vi "Client_Init.vi"(0 "object in":refnum<class "Client.lvclass">, 2 "File Type":T2, 3 "File Method":T1, 5 "Error In":errorcluster) -> (14 "object out":refnum<class "Client.lvclass">, 19 "Error Out":errorcluster)   [LabVIEW 2024, in "Client.lvclass"]
uses:
  Client.lvclass
  Support/Type Def/File Type.ctl
  Support/Type Def/File Method.ctl
  Implementations/Logger/Logger.lvclass
  Implementations/Viewer/Viewer.lvclass
  Abstractions/Excel/Excel.lvclass
  Abstractions/TDMS/TDMS.lvclass
  Client.lvclass/Client.ctl
  <vilib>/Utility/file.llb/Write Delimited Spreadsheet (string).vi
  IDataMethod_interface/IDataMethod.lvclass
  Abstractions/DataType/DataType.lvclass
panel:
  # "Connector Pane"
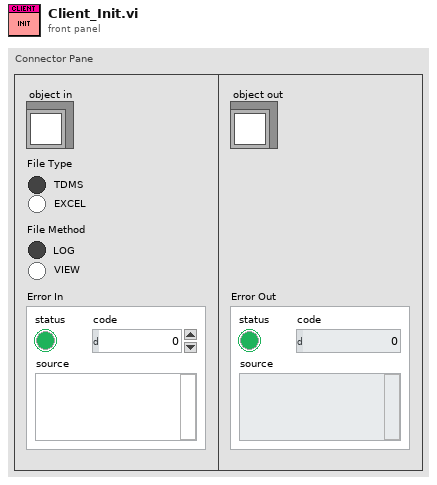
[diagram p1: front panel]
types:
  T1 = typedef "File Method.ctl" = enum32{"Log", "View"}
  T2 = typedef "File Type.ctl" = enum32{"TDMS", "EXCEL"}
  T3 = enum16{"open", "open or create", "create or replace", "create", "open (read-only)"}
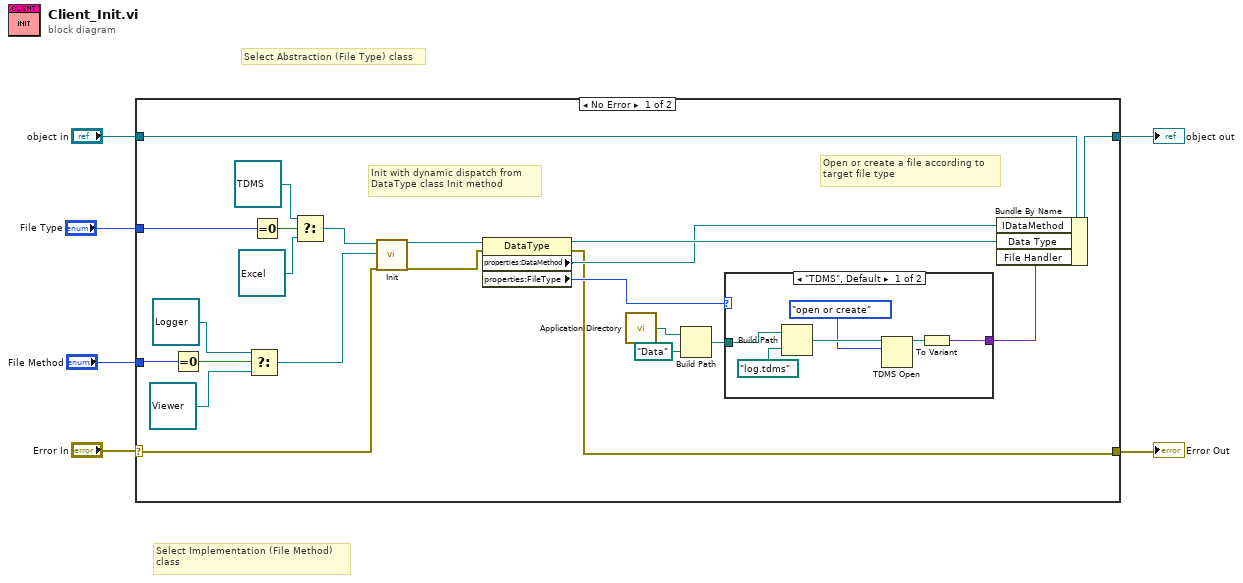
[diagram p0: block diagram]
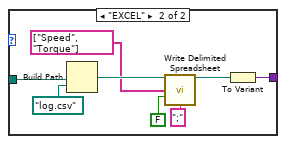
[diagram p2: hidden frame]
diagram:
  # "Select Abstraction (File Type) class"
  # "Select Implementation (File Method)\nclass"
  n1 = case shown="No Error" "Error In" {
    selector: "Error In" -> [w10 w44]
    tunnel: "object in" -> [w29 w45]
    tunnel: [w28 w45] -> w5
    tunnel: [w20 w44] -> w3
    tunnel: "File Method" -> [w19 _]
    tunnel: "File Type" -> [w16 _]
    frame No Error {
      # "Open or create a file according to\ntarget file type"
      # "Init with dynamic dispatch from\nDataType class Init method"
      n2 = Equal To 0?(x=w19) -> (x = 0?=w18:bool)
      n3 = Select(t=refnum<class "Logger.lvclass"> refnum ("Logger"), s=w18, f=refnum<class "Viewer.lvclass"> refnum ("Viewer")) -> (s? t:f=w11:refnum<class "IDataMethod.lvclass">)
      n4 = Equal To 0?(x=w16) -> (x = 0?=w17:bool)
      n5 = Select(t=refnum<class "TDMS.lvclass"> refnum ("TDMS"), s=w17, f=refnum<class "Excel.lvclass"> refnum ("Excel")) -> (s? t:f=w12:refnum<class "DataType.lvclass">)
      n6 = call-dynamic "Init.vi"("object in"=w12, "Data Method"=w11, "error in (no error)"=w10) -> ("object out"=w8:refnum<class "DataType.lvclass">, "error out"=w9:errorcluster)  [unwired: 15 in]
      n7 = property class="DataType"(reference=w8, error in=w9) -> (reference out=w23:refnum<class "DataType.lvclass">, error out=w20:errorcluster, "properties:DataMethod"=w22:refnum<class "IDataMethod.lvclass">, "properties:FileType"=w21:T2)
      n8 = call <vilib>:"Application Directory.vi"() -> ("Application Directory"=w25:path)
      n9 = Build Path(base path=w25, name or relative path=path "Data") -> (appended path=w27:path)
      n10 = case shown="\"TDMS\", Default" w21 {
        tunnel: w27 -> [w35 w42]
        tunnel: [w30 w36] -> w24
        frame "TDMS", Default {
          n11 = Build Path(base path=w35, name or relative path=path "log.tdms") -> (appended path=w34:path)
          n12 = TDMS Open(10:T3."open or create" ("operation (0:open)"), 11:w34) -> (3:w31:refnum<k34>)  [unwired: 5 in, 1 out]
          n13 = To Variant(anything=w31) -> (Variant=w30:variant)
        }
        frame "EXCEL" {
          n14 = Build Path(base path=w42, name or relative path=path "log.csv") -> (appended path=w40:path)
          n15 = call-poly <vilib>:"Write Delimited Spreadsheet.vi"("file path (dialog if empty)"=w40, "1D data"=string[] ["Speed", "Torque"], "append to file? (new file:F)"=FALSE, "delimiter (\\t)"=";" ("delimiter (\\t)")) -> ("new file path (Not A Path if cancelled)"=w43:path)  [unwired: 10 in, 1 out]
          n16 = To Variant(anything=w43) -> (Variant=w36:variant)
        }
      }
      n17 = Bundle By Name(cluster=w29, "IDataMethod"=w22, "Data Type"=w23, "File Handler"=w24) -> (w28:refnum<class "Client.lvclass">)
    }
    frame Error {
    }
  }
  "object out" <- w5
  "Error Out" <- w3
